vi "Instr_InitObject.vi"(8 "error in (no error)":errorcluster, 9 "Instrument Configuration":variant, 10 "Instrument address":refnum<visa-resource-name>, 11 "InstrControl in":refnum<class "InstrControl.lvclass">) -> (0 "error out":errorcluster, 3 "InstrControl out":refnum<class "InstrControl.lvclass">)   [LabVIEW 2018, in "InstrControl.lvclass"]
uses:
  InstrControl.lvclass
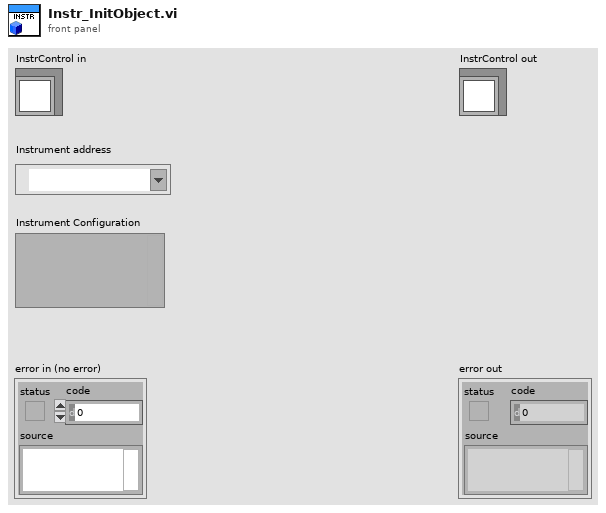
[diagram p1: front panel]
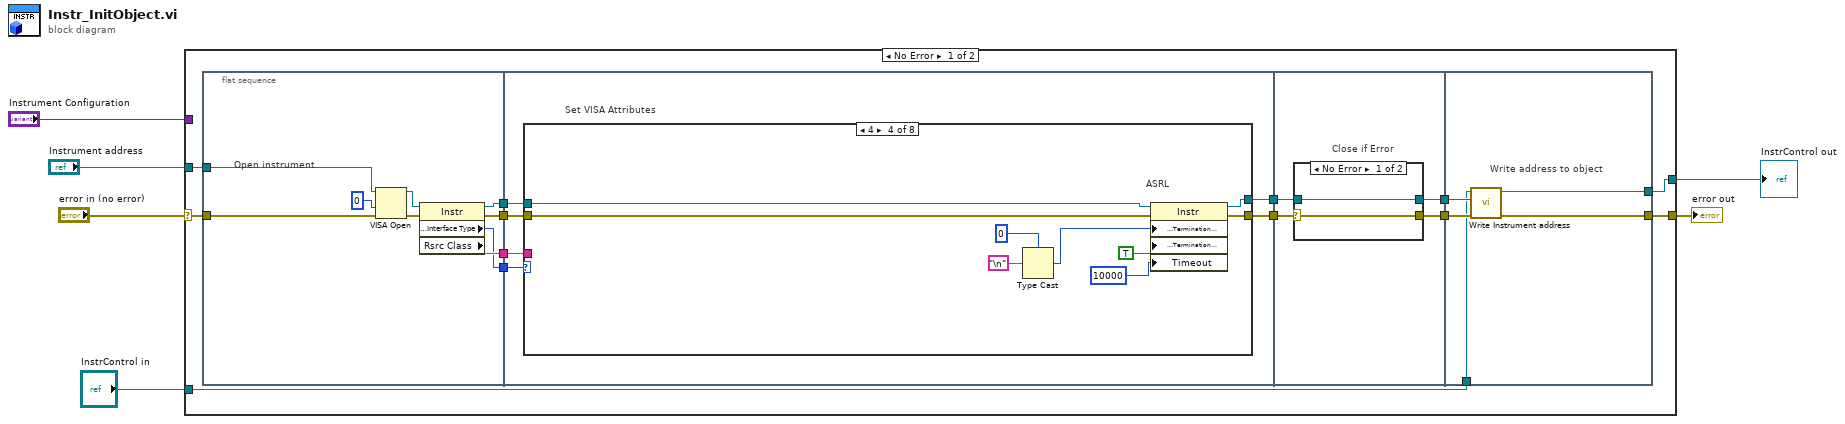
[diagram p0: block diagram]
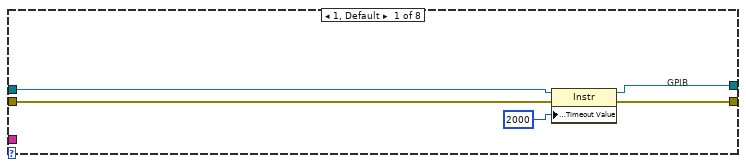
[diagram p2: hidden frame]
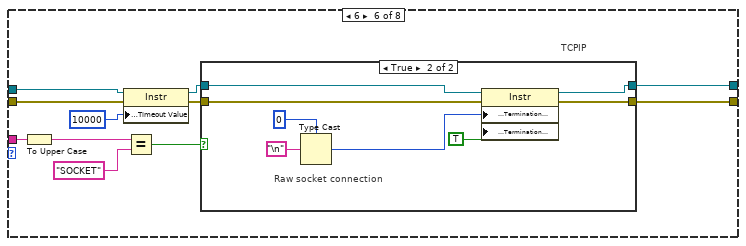
[diagram p6: hidden frame]
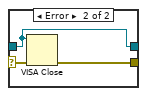
[diagram p10: hidden frame]
diagram:
  n1 = case shown="No Error" "error in (no error)" {
    selector: "error in (no error)" -> [w15 w85]
    tunnel: [w11 w85] -> w5
    tunnel: [w8 w84] -> w3
    tunnel: "InstrControl in" -> [w7 w84]
    tunnel: "Instrument address" -> [w19 _]
    tunnel: "Instrument Configuration" -> [_ _]
    frame No Error {
      n2 = flat-sequence {
        tunnel: w19 -> [w25]
        tunnel: [w24] -> w18
        tunnel: [w23] -> w17
        tunnel: [w22] -> w16
        tunnel: w15 -> [w21]
        tunnel: [w20] -> w14
        tunnel: w18 -> [w34]
        tunnel: w17 -> [w33]
        tunnel: w16 -> [w32]
        tunnel: w14 -> [w31]
        tunnel: [w30] -> w13
        tunnel: [w29] -> w12
        tunnel: w13 -> [w73]
        tunnel: w12 -> [w72]
        tunnel: [w71] -> w10
        tunnel: [w70] -> w9
        tunnel: [w82] -> w11
        tunnel: w10 -> [w83]
        tunnel: w9 -> [w81]
        tunnel: [w80] -> w8
        tunnel: w7 -> [w79]
        frame #0 {
          # "Open instrument"
          n3 = VISA Open(access mode=u32 0, error in (no error)=w21, VISA resource name=w25) -> (VISA resource name=w27:refnum<visa-resource-name>, error out=w28:errorcluster)  [unwired: 2 out]
          n4 = property class="Instr"(reference=w27, error in=w28) -> (reference out=w24:refnum<visa-resource-name>, error out=w20:errorcluster, "Interface Information:Interface Type"=w22:u16, "Rsrc Class"=w23:string)
        }
        frame #1 {
          # "Set VISA Attributes"
          n5 = case shown="4" w32 {
            tunnel: [w37 _ _ w47 _ w59 _ _] -> w29
            tunnel: [w36 _ _ w46 _ w58 _ _] -> w30
            tunnel: w34 -> [w39 _ _ w45 _ w52 _ _]
            tunnel: w31 -> [w38 _ _ w48 _ w50 _ _]
            tunnel: w33 -> [_ _ _ _ _ w57 _ _]
            frame 1, Default {
              # "GPIB"
              n6 = property class="Instr"(reference=w39, error in=w38, "General Settings:Timeout Value"=u32 2000) -> (reference out=w37:refnum<visa-resource-name>, error out=w36:errorcluster)
            }
            frame 2 {
              # "don't have any instrument with this\nanyone happy to fill this in?"
              # "VXI"
            }
            frame 3 {
              # "don't have any instrument with this\nanyone happy to fill this in?"
              # "GPIB-VXI"
            }
            frame 4 {
              # "ASRL"
              n7 = Type Cast(type=u8 0, x="\n") -> (*(type *) &x=w41:u8)
              n8 = property class="Instr"(reference=w45, error in=w48, "Message Based Settings:Termination Character"=w41, "Message Based Settings:Termination Character Enable"=TRUE, "Timeout"=u32 10000 ("General Settings:Timeout Value")) -> (reference out=w47:refnum<visa-resource-name>, error out=w46:errorcluster)
            }
            frame 5 {
              # "don't have any instrument with this\nanyone happy to fill this in?"
              # "PXI"
            }
            frame 6 {
              # "TCPIP"
              n9 = To Upper Case(1:w57) -> (0:w56:string)
              n10 = property class="Instr"(reference=w52, error in=w50, "General Settings:Timeout Value"=u32 10000) -> (reference out=w51:refnum<visa-resource-name>, error out=w49:errorcluster)
              n11 = Equal?(x=w56, y="SOCKET" ("regular expression")) -> (x = y?=w54:bool)
              n12 = case shown="True" w54 {
                tunnel: w49 -> [w60 w69]
                tunnel: [w61 w68] -> w59
                tunnel: [w60 w67] -> w58
                tunnel: w51 -> [w61 w62]
                frame False {
                  # "VXI-11 connection"
                }
                frame True {
                  # "Raw socket connection"
                  n13 = Type Cast(type=u8 0, x="\n") -> (*(type *) &x=w63:u8)
                  n14 = property class="Instr"(reference=w62, error in=w69, "Message Based Settings:Termination Character"=w63, "Message Based Settings:Termination Character Enable"=TRUE) -> (reference out=w68:refnum<visa-resource-name>, error out=w67:errorcluster)
                }
              }
            }
            frame 7 {
              # "USB"
              # "don't have any instrument with this\nanyone happy to fill this in?"
            }
            frame 9 {
              # "FireWire"
              # "don't have any instrument with this\nanyone happy to fill this in?"
            }
          }
        }
        frame #2 {
          # "Close if Error"
          n15 = case shown="No Error" w73 {
            selector: w73 -> [w75 w78]
            tunnel: w72 -> [w74 w76]
            tunnel: [w75 w77] -> w71
            tunnel: [w74 w76] -> w70
            frame No Error {
            }
            frame Error {
              n16 = VISA Close(VISA resource name=w76, error in (no error)=w78) -> (error out=w77:errorcluster)
            }
          }
        }
        frame #3 {
          # "Write address to object"
          n17 = call-dynamic "Write Instrument address.vi"("error in (no error)"=w83, "GPIB address"=w81, "InstControl in"=w79) -> ("error out"=w82:errorcluster, "InstControl out"=w80:refnum<class "InstrControl.lvclass">)  [unwired: 7 in]
        }
      }
    }
    frame Error {
    }
  }
  "error out" <- w5
  "InstrControl out" <- w3
